vi "Demo.vi"() -> ()   [LabVIEW 2013]
panel:
  out "OldName":string
  out "OldFullPath":string
  out "Name":string
  out "ChangeType":i32(ring)=1 items=["Created"=1, "Deleted"=2, "Changed"=4, "Renamed"=8, "All"=15]
  out "FullPath":string
  in  "Folder Path":path
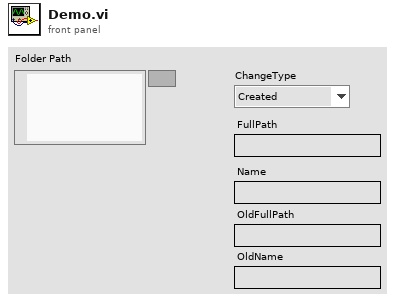
[diagram p1: front panel]
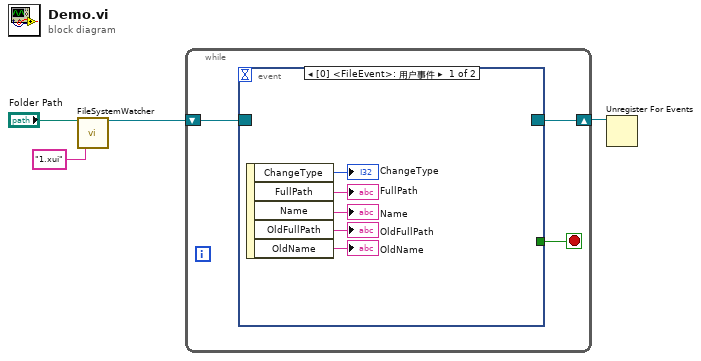
[diagram p0: block diagram]
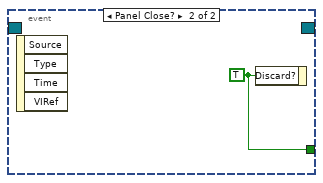
[diagram p2: hidden frame]
diagram:
  n1 = call "FileSystemWatcher.vi"("Folder Path"="Folder Path", "Filter"="1.xui") -> ("RegEvent"=w4:refnum<event-registration>)  [unwired: 16 in, 1 out]
  n2 = while {
    shift-right: [w6] -> w3
    shift-left: w4 -> [w7]
    stop <- w5 stop-if-true
    n3 = event shown="[0] <FileEvent>: 用户事件" {
      selector: w7 -> [_ _]
      dyn-events: [_ _] -> w6
      timeout: _ -> [_ _]
      tunnel: [_ w13] -> w5
      event User Event {
        n4 = event-data() -> ("ChangeType"=→"ChangeType":i32, "FullPath"=→"FullPath":string, "Name"=→"Name":string, "OldFullPath"=→"OldFullPath":string, "OldName"=→"OldName":string)  [unwired: 1 in]
      }
      event Panel Close? {
        w13 = TRUE ("放弃？")
        n5 = event-data() -> ()  [unwired: 1 in, 4 out]
        n6 = event-data("Discard?"=w13) -> ()  [unwired: 1 in, 1 out]
      }
    }
  }
  n7 = Unregister For Events(event registration refnum=w3) -> ()  [unwired: 1 in, 1 out]
